vi "Accelerometer.vi"() -> ()   [LabVIEW 2010]
uses:
  <vilib>/eio/EIONode/EIONode.xnode
  <vilib>/rvi/eio/nirviEIOImplementation/nirviEIOImplementation.xnode
  <vilib>/rvi/eio/common/nirviEmuClasses.ctl
  <vilib>/rvi/DataTransferAndStorage/Container/XNode/niFpgaContainer.xnode
  <vilib>/rvi/eio/common/nirviEmuTemplateMethod_noerrors.vi
  <vilib>/rvi/FIFO/Fifo_Resource/nirvififoEmulationSetSize.vi
  <vilib>/rvi/DataTransferAndStorage/Container/Common/niFpgaContainerGetUniqueNameForEmu.vi
panel:
  out "Y Acceleration":fxp<+/-,24,4> format="%.22g"
  out "Terminate":bool
  in  "Acceleration Threshold":fxp<+/-,24,4> format="%.22g"
  in  "Fan Speed Control":fxp<+/-,20,5> format="%_6g"
  out "Threshold Exceeded?":bool
  in  "Stop":bool
  in  "Sample Period (us)":u32
  out "Overflow Occurred?":bool
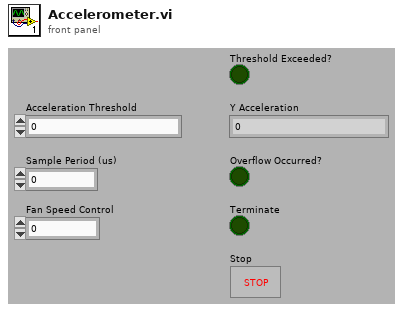
[diagram p1: front panel]
types:
  T1 = typedef "nirviEmuClasses.ctl" = enum16{"IO Read", "IO Write", "Method", "Property Read", "Property Write"}
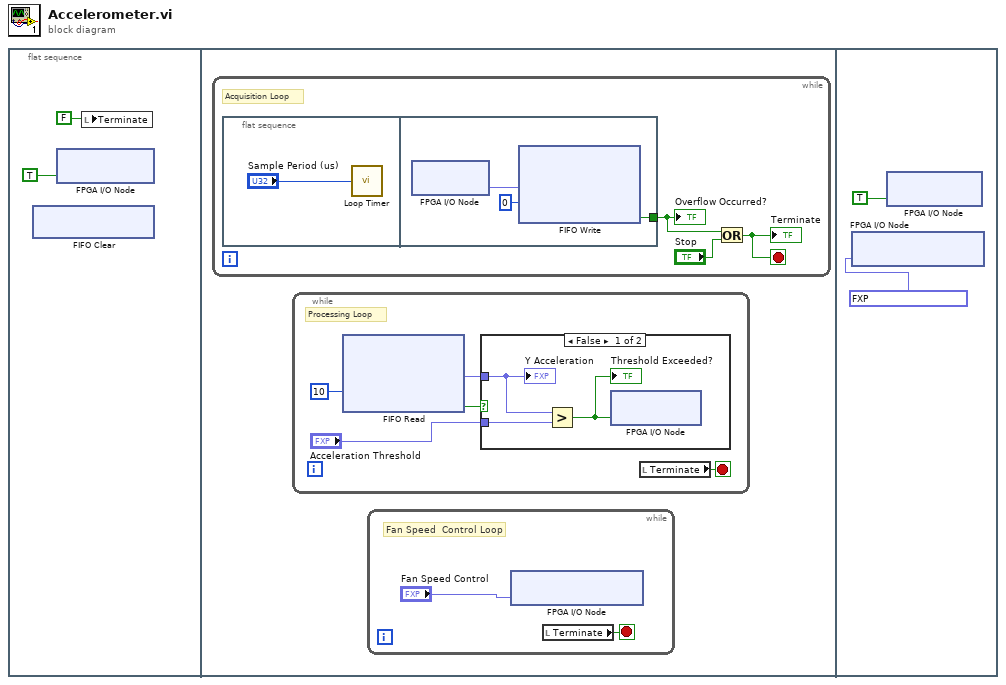
[diagram p0: block diagram]
diagram:
  n1 = flat-sequence {
    frame #0 {
      n2 = xnode "FIFO Clear"() -> ()  [unwired: 1 in, 1 out]
      n3 = xnode "FPGA I/O Node"("Mod2/Start"=TRUE) -> ()  [unwired: 1 in, 1 out]
      n4 = local write "Terminate"(FALSE ("Terminate 2")) -> ()
    }
    frame #1 {
      n5 = while {
        stop <- w136 stop-if-true
        # "Acquisition Loop"
        n6 = flat-sequence {
          tunnel: [w142] -> w137
          frame #0 {
            n7 = call "Loop Timer"("Count(uSec)"="Sample Period (us)") -> ()  [unwired: 1 out]
          }
          frame #1 {
            n8 = xnode "FPGA I/O Node"() -> ("Y Accel"=w140:fxp<+/-,24,4>)  [unwired: 1 in, 1 out]
            n9 = xnode ("FIFO Write")("Element"=w140, "Timeout"=0) -> ("Timed Out?"=w142:bool)  [unwired: 1 in, 1 out]
          }
        }
        n10 = Or(x=w137, y="Stop") -> (x .or. y?=w136:bool)
        "Terminate" <- w136
        "Overflow Occurred?" <- w137
      }
      n11 = while {
        stop <- w70 stop-if-true
        # "Processing Loop"
        n12 = xnode ("FIFO Read")("Timeout"=10) -> ("Element"=w68:fxp<+/-,24,4>, "Timed Out?"=w67:bool)  [unwired: 1 in, 1 out]
        n13 = case shown="False" w67 {
          tunnel: w68 -> [w72 _]
          tunnel: "Acceleration Threshold" -> [w71 _]
          frame False {
            n14 = Greater?(x=w72, y=w71) -> (0:w73:bool)
            "Threshold Exceeded?" <- w73
            n15 = xnode "FPGA I/O Node"("FPGA LED"=w73) -> ()  [unwired: 1 in, 1 out]
            "Y Acceleration" <- w72
          }
          frame True {
          }
        }
        n16 = local read "Terminate"() -> (w70:bool)
      }
      n17 = while {
        stop <- w54 stop-if-true
        # "Fan Speed  Control Loop"
        n18 = xnode "FPGA I/O Node"("Fan Speed Control"="Fan Speed Control") -> ()  [unwired: 1 in, 1 out]
        n19 = local read "Terminate"() -> (w54:bool)
      }
    }
    frame #2 {
      n20 = xnode "FPGA I/O Node"("Fan Speed Control"=fxp<+/-,20,5> 0.0) -> ()  [unwired: 1 in, 1 out]
      n21 = xnode "FPGA I/O Node"("Mod2/Stop"=TRUE ("Mod2/Start")) -> ()  [unwired: 1 in, 1 out]
    }
  }
